vi "VISA Write Read.vi"(8 "error in (no error)":errorcluster, 10 "8800 Command":string, 11 "VISA Refnum in":refnum<visa-resource-name>) -> (0 "error out":errorcluster, 2 "read buffer":string, 3 "VISA Refnum out":refnum<visa-resource-name>)   [LabVIEW 2023, in "Thermotron 8800.lvlib"]
doc: "Write string command message using VISA to 8800 and read back response"
uses:
  Thermotron 8800.lvlib
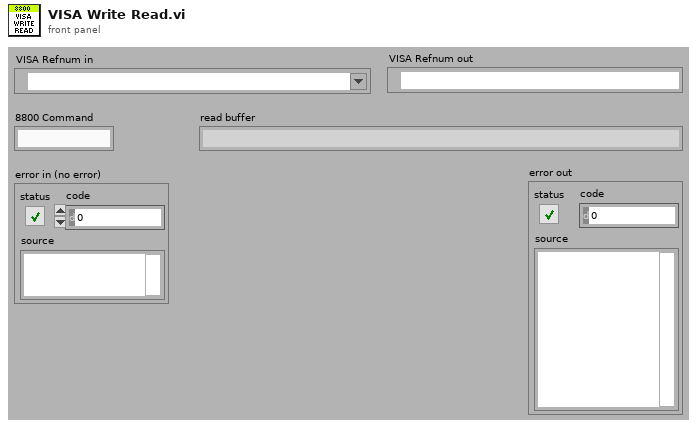
[diagram p1: front panel]
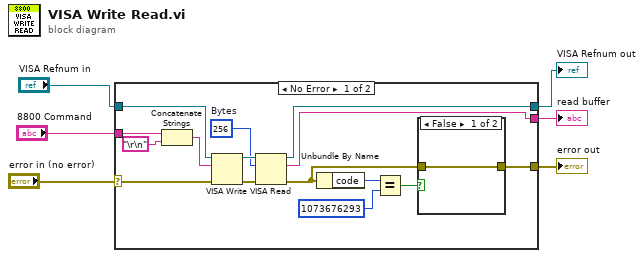
[diagram p0: block diagram]
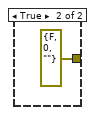
[diagram p2: hidden frame]
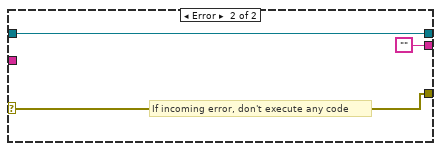
[diagram p3: hidden frame]
diagram:
  n1 = case shown="No Error" "error in (no error)" {
    selector: "error in (no error)" -> [w14 w24]
    tunnel: "8800 Command" -> [w15 _]
    tunnel: [w13 w24] -> w1
    tunnel: "VISA Refnum in" -> [w12 w26]
    tunnel: [w11 w26] -> w3
    tunnel: [w10 ""] -> w2
    frame No Error {
      w7 = u32 256  # Bytes
      n2 = Concatenate Strings(w15, "\r\n") -> (w17:string)
      n3 = VISA Write(VISA resource name=w12, write buffer=w17, error in (no error)=w14) -> (VISA resource name out=w9:refnum<visa-resource-name>, error out=w8:errorcluster)  [unwired: 1 out]
      n4 = VISA Read(VISA resource name=w9, byte count=w7, error in (no error)=w8) -> (VISA resource name out=w11:refnum<visa-resource-name>, read buffer=w10:string, error out=w21:errorcluster)  [unwired: 1 out]
      n5 = Unbundle By Name(w21) -> ("code"=w18:i32)
      n6 = Equal?(x=w18, y=1073676293) -> (x = y?=w20:bool)
      n7 = case shown="False" w20 {
        tunnel: w21 -> [w22 _]
        tunnel: [w22 errorcluster {"status"=FALSE, "code"=0, "source"=""} ("error out")] -> w13
        frame False {
        }
        frame True {
        }
      }
    }
    frame Error {
      # "If incoming error, don't execute any code"
    }
  }
  "error out" <- w1
  "VISA Refnum out" <- w3
  "read buffer" <- w2
